vi "Reinitialize Control Values to Default.vi"(8 "error in":errorcluster, 11 "VI Ref":refnum<vi>) -> (0 "error out":errorcluster)   [LabVIEW 2025]
panel:
  out "Array":string[](array[string])
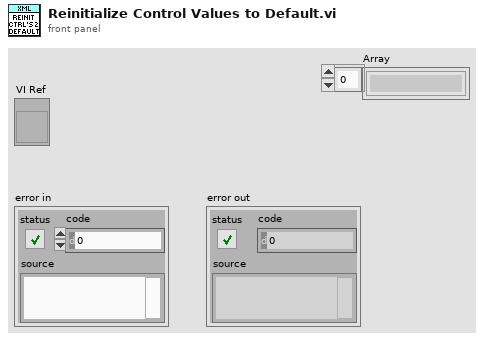
[diagram p1: front panel]
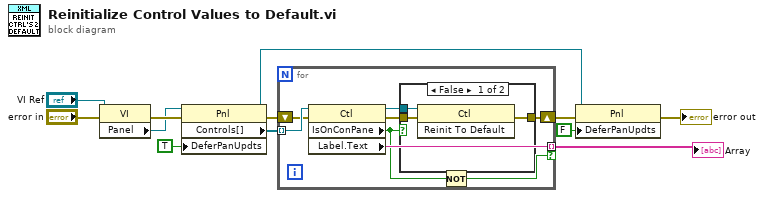
[diagram p0: block diagram]
diagram:
  n1 = property class="VI"(reference="VI Ref", error in="error in") -> (error out=w11:errorcluster, "Panel"=w6:refnum<vi>)  [unwired: 1 out]
  n2 = property class="Pnl"(reference=w6, error in=w11, "DeferPanUpdts"=TRUE ("Defer Panel Updates")) -> (reference out=w3:refnum<vi>, error out=w8:errorcluster, "Controls[]"=w12:refnum<vi>[])
  n3 = for {
    tunnel: w12 -> [w18] mode=indexing
    shift-right: [w20] -> w4
    shift-left: w8 -> [w17]
    tunnel: [w15] -> w7 mode=indexing if=w13
    n4 = property class="Ctl"(reference=w18, error in=w17) -> (reference out=w19:refnum<vi>, error out=w16:errorcluster, "IsOnConPane"=w14:bool, "Label.Text"=w15:string)
    n5 = case shown="False" w14 {
      tunnel: [w23 w24] -> w20
      tunnel: w19 -> [w22 _]
      tunnel: w16 -> [w21 w24]
      frame False {
        n6 = invoke class="Ctl" method="Reinit To Default"(reference=w22, error in=w21) -> (error out=w23:errorcluster)  [unwired: 1 in, 2 out]
      }
      frame True {
      }
    }
    n7 = Not(x=w14) -> (.not. x?=w13:bool)
  }
  "Array" <- w7
  n8 = property class="Pnl"(reference=w3, error in=w4, "DeferPanUpdts"=FALSE ("Defer Panel Updates")) -> (error out=→"error out":errorcluster)  [unwired: 1 out]
